vi "Start Create Procedure.vi"(8 "에러 입력(에러 없음)":errorcluster, 9 "Model List":refnum<vi>[](array[refnum]), 10 "세부분류코드":string, 11 "CMC":refnum<vi>) -> (0 "에러 출력":errorcluster, 3 "Calfunc":string[][](array[string]), 4 "Data":string[][](array[string]), 5 "CMC":string[][](array[string]), 6 "모델정보 배열":string[][](array[string]), 7 "모델 및 옵션":string[][](array[string]))   [LabVIEW 2020]
uses:
  Support/Controls/Clst_Query Info.ctl
  Support/Controls/Cmd_Read Query.ctl
  Support/Public/Polymorph/Array Dedup_2D Str.vi
  Support/Public/Polymorph/Cell Space_Table.vi
  Support/Public/Polymorph/Array Dedup_1D Str.vi
  Support/Public/Polymorph/Data Class_2D Str.vi
  <vilib>/addons/database/NI_Database_API.lvlib
panel:
  out "Func List":string[](array[string])
  # "DSEQ\nCLSMAN_EXT\nFUNC\nFUNC_EXT\nC1_LOW\nC1_LUNIT\nC1_LCON\nC1_HIGH\nC1_HUNIT\nC1_HCON\nRANGE_LOW\nRANGE_LUNIT\nRANGE_LDIV\nRANGE_HIGH\nRANGE_HUNIT\nRANGE_HDIV"
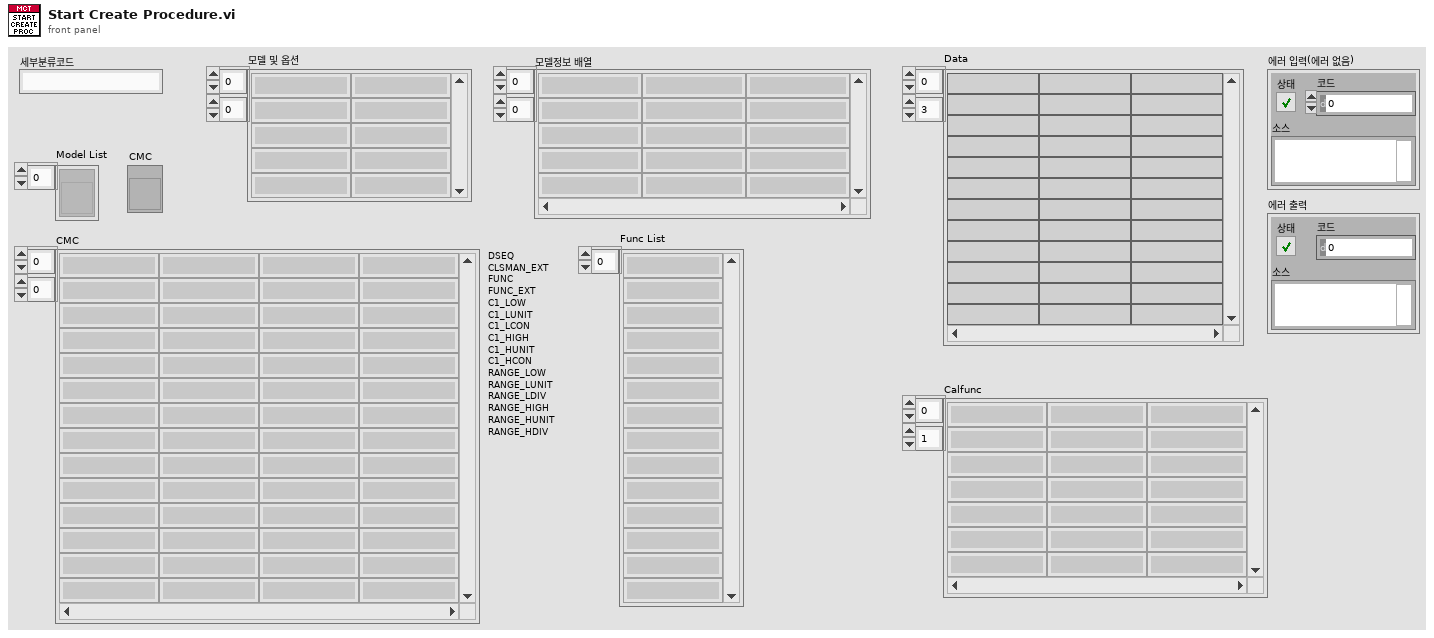
[diagram p1: front panel]
types:
  T1 = typedef "Cmd_Read Query.ctl" = enum16{"교정자 이름 얻기", "인증교정자 얻기", "기술책임자 얻기", "기책부책 얻기", "등록번호 얻기", "등록정보 얻기", "업체정보 얻기", "교정일자(CAMAS) 얻기", "교정일자(CALSTD) 얻기", "교정환경 얻기", "교정절차서 목록 얻기", "교정절차서명 얻기", "교정절차 목록얻기", "교정절차 얻기", "PROC 교정절차 얻기", "PROC SPEC 얻기", "교정절차(Func별) 얻기", "교정절차(Func_ext별) 얻기", "기관코드 얻기", "교정기능(세부분류) 얻기", "교정기능(모델) 얻기", "교정기능 목록 얻기", "교정기능 명칭 얻기", "교정기능 항목명칭 얻기", "DB (사용기준기) 얻기", "DB (기준기이름) 얻기", "DB (기준기이름목록) 얻기", "DB (기준기목록) 얻기", "DB (기준기값) 얻기", "DB (CMC) 얻기", "DB (FUNC) 얻기", "DB (CALNAME) 얻기", "DB (STDNAME) 얻기", "DB (SPEC) 얻기", "모델(항목전체) 얻기", "모델(최대범위) 얻기", "모델(최소범위) 얻기", "모델(최대최소) 얻기", "모델(범위조건) 얻기", "모델(등록요청) 얻기", "모델(형식별) 얻기", "모델(조건별) 얻기", "모델(모델검색) 얻기", "세부분류 목록 얻기", "기준기등록리스트 얻기", "STD Cal Date Check", "DB등록일자 얻기", "적용항목 얻기", "기타정보 얻기", "기준기요청 얻기", "서버버전 얻기"}
  T2 = typedef "Clst_Query Info.ctl" = cluster{"사번":string, "등록번호":string, "업체명":string, "세부분류코드":string, "형식":string, "기기번호":string, "FUNC":string, "FUNC_EXT":string, "옵션":string, "추가문자열":string, "일자":string, "배열 1":string[], "배열 2":string[], "항목명":string, "문자열":string, "이름":string}
  T3 = typedef "NI_Database_API.lvlib/Conn ObjectReference.ctl" = refnum<k1>
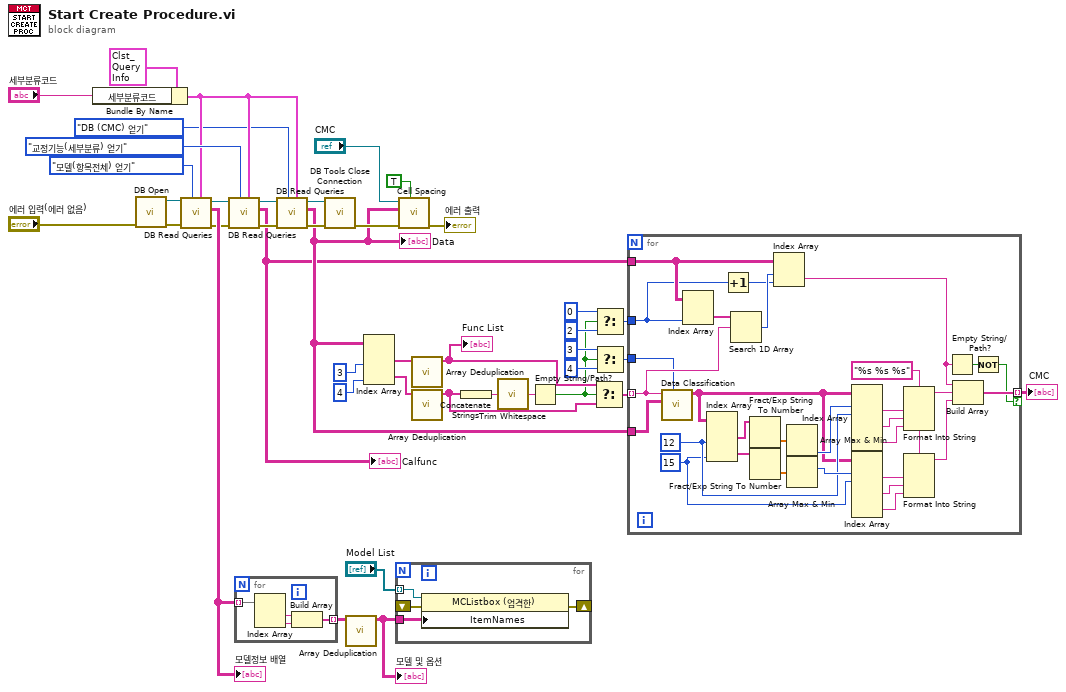
[diagram p0: block diagram]
diagram:
  n1 = Bundle By Name(cluster=T2 {"사번"="", "등록번호"="", "업체명"="", "세부분류코드"="", "형식"="", "기기번호"="", "FUNC"="", "FUNC_EXT"="", "옵션"="", "추가문자열"="", "일자"="", "배열 1"=[], "배열 2"=[], "항목명"="", "문자열"="", "이름"=""} ("Query info"), "세부분류코드"="세부분류코드") -> (w38:T2)
  n2 = call "DB Open.vi"("에러 입력"="에러 입력(에러 없음)") -> ("에러 출력"=w36:errorcluster, "참조 번호 출력"=w35:T3)  [unwired: 9 in]
  n3 = call "DB Read Queries.vi"("Query info"=w38, "Query Command"=Cmd_Read_Query."모델(항목전체) 얻기", "에러 입력(에러 없음)"=w36, "참조 번호 입력"=w35) -> ("에러 출력"=w17:errorcluster, "Data"=w32:string[][], "참조 번호 출력"=w26:T3)  [unwired: 3 in, 2 out]
  "모델정보 배열" <- w32
  n4 = call "DB Read Queries.vi"("Query info"=w38, "Query Command"=Cmd_Read_Query."교정기능(세부분류) 얻기", "에러 입력(에러 없음)"=w17, "참조 번호 입력"=w26) -> ("에러 출력"=w37:errorcluster, "Data"=w14:string[][], "참조 번호 출력"=w34:T3)  [unwired: 3 in, 2 out]
  "Calfunc" <- w14
  n5 = for {
    tunnel: w32 -> [w46] mode=indexing
    tunnel: [w44] -> w31 mode=indexing
    n6 = Index Array(array=w46) -> (element #1=w45:string, element #2=w43:string)  [unwired: 2 in]
    n7 = Build Array(w45, w43) -> (w44:string[])
  }
  n8 = call "DB Read Queries.vi"("Query info"=w38, "Query Command"=Cmd_Read_Query."DB (CMC) 얻기", "에러 입력(에러 없음)"=w37, "참조 번호 입력"=w34) -> ("에러 출력"=w23:errorcluster, "Data"=w19:string[][], "참조 번호 출력"=w40:T3)  [unwired: 3 in, 2 out]
  "Data" <- w19
  n9 = call <vilib>:"DB Tools Close Connection.vi"("error in (no error)"=w23, "connection reference"=w40) -> ("error out"=w22:errorcluster)  [unwired: 5 in]
  n10 = call-poly "Array Deduplication.vi"("배열 in"=w31) -> ("배열 out"=w30:string[][])  [unwired: 9 in, 1 out]
  "모델 및 옵션" <- w30
  n11 = Index Array(array=w19, index (col) #1=3 ("비활성화된 인덱스 (열)"), index (col) #2=4 ("비활성화된 인덱스 (열)")) -> (element #1=w28:string[], element #2=w15:string[])  [unwired: 2 in]
  n12 = for {
    tunnel: "Model List" -> [w50] mode=indexing
    tunnel: w30 -> [w47]
    shift-right: [w49] -> _
    shift-left: _ -> [w48]
    n13 = property on="프로퍼티 노드" class="MCListbox (엄격한)"(reference=w50, error in=w48, "ItemNames"=w47) -> (error out=w49:errorcluster)  [unwired: 1 out]
  }
  n14 = call-poly "Cell Spacing.vi"("빈내용 숨기기?(F)"=TRUE, "error in"=w22, "Data in"=w19, "테이블 참조 in"="CMC") -> ("error out"=→"에러 출력":errorcluster)  [unwired: 5 in, 2 out]
  n15 = call-poly "Array Deduplication.vi"("배열 in"=w28) -> ("배열 out"=w11:string[])  [unwired: 9 in, 1 out]
  "Func List" <- w11
  n16 = call-poly "Array Deduplication.vi"("배열 in"=w15) -> ("배열 out"=w9:string[])  [unwired: 9 in, 1 out]
  n17 = Concatenate Strings(w9) -> (w13:string)
  n18 = call <vilib>:"Trim Whitespace.vi"("string"=w13) -> ("trimmed string"=w12:string)  [unwired: 1 in]
  n19 = Empty String/Path?(string/path=w12) -> (empty?=w2:bool)
  n20 = Select(t=w11, s=w2, f=w9) -> (s? t:f=w10:string[])
  n21 = Select(t=0 ("비활성화된 인덱스 (열)"), s=w2, f=2 ("비활성화된 인덱스 (열)")) -> (s? t:f=w4:i32)
  n22 = Select(t=3 ("비활성화된 인덱스 (열)"), s=w2, f=4 ("비활성화된 인덱스 (열)")) -> (s? t:f=w7:i32)
  n23 = for {
    tunnel: w10 -> [w59] mode=indexing
    tunnel: w19 -> [w80]
    tunnel: [w78] -> w18 mode=indexing if=w53
    tunnel: w14 -> [w58]
    tunnel: w7 -> [w56]
    tunnel: w4 -> [w51]
    w63 = 15 ("비활성화된 인덱스 (열)")
    w67 = 12 ("비활성화된 인덱스 (열)")
    w75 = "%s %s %s" ("포맷 문자열")
    n24 = call-poly "Data Classification.vi"("인덱스"=w56, "DATA 입력"=w80, "검색 문자열"=w59) -> ("DATA 출력"=w64:string[][])  [unwired: 4 in, 4 out]
    n25 = Index Array(array=w58, index (col)=w51) -> (element=w60:string[])  [unwired: 1 in]
    n26 = Index Array(array=w64, index (col) #1=w67, index (col) #2=w63) -> (element #1=w70:string[], element #2=w69:string[])  [unwired: 2 in]
    n27 = Increment(x=w51) -> (x+1=w52:i32)
    n28 = Search 1D Array(1D array=w60, element=w59) -> (index of element=w57:i32)  [unwired: 1 in]
    n29 = Fract/Exp String To Number(string=w70) -> (number=w72:dbl[])  [unwired: 3 in, 1 out]
    n30 = Fract/Exp String To Number(string=w69) -> (number=w71:dbl[])  [unwired: 3 in, 1 out]
    n31 = Index Array(array=w58, index (row)=w57, index (col)=w52) -> (element=w55:string)
    n32 = Array Max & Min(array=w72) -> (min index (indices)=w68:i32)  [unwired: 3 out]
    n33 = Array Max & Min(array=w71) -> (max index (indices)=w73:i32)  [unwired: 3 out]
    n34 = Index Array(array=w64, index (row) #1=w68, index (col) #1=w67) -> (element #1=w79:string, element #2=w66:string, element #3=w65:string)  [unwired: 4 in]
    n35 = Index Array(array=w64, index (row) #1=w73, index (col) #1=w63) -> (element #1=w76:string, element #2=w62:string, element #3=w61:string)  [unwired: 4 in]
    n36 = Format Into String(format string=w75, w79, w66, w65) -> (resulting string=w77:string)  [unwired: 2 in, 1 out]
    n37 = Format Into String(format string=w75, w76, w62, w61) -> (resulting string=w74:string)  [unwired: 2 in, 1 out]
    n38 = Empty String/Path?(string/path=w55) -> (empty?=w54:bool)
    n39 = Build Array(w55, w77, w74) -> (w78:string[])
    n40 = Not(x=w54) -> (.not. x?=w53:bool)
  }
  "CMC" <- w18
